vi "Lang Set Desc i.vi"(8 "error in (no error)":errorcluster, 10 "i":T1, 11 "LF2R IDE in":refnum<class "Main Panel.lvclass">) -> (0 "error out":errorcluster, 3 "LF2R IDE out":refnum<class "Main Panel.lvclass">)   [LabVIEW 2018, in "Framework.lvlib" / "Framework.lvclass"]
uses:
  Framework/Framework/Framework.lvclass
  Main Panel.lvclass
  D:/project/hobby/LabVIEW/LF2R/LabVIEW/Source/Actor/Framework/Framework/Framework.lvclass
  C:/Program Files (x86)/National Instruments/LabVIEW 2018/vi.lib/MGI/Panel Manager/Panel Actor/Panel Actor/Panel Actor.lvclass
  C:/Program Files (x86)/National Instruments/LabVIEW 2018/vi.lib/MGI/Monitored Actor/Monitored Actor/Monitored Actor/Monitored Actor.lvclass
  C:/Program Files (x86)/National Instruments/LabVIEW 2018/vi.lib/ActorFramework/Actor/Actor.lvclass
  Const Lang Property.ctl
  Const UI Desc Frame i.ctl
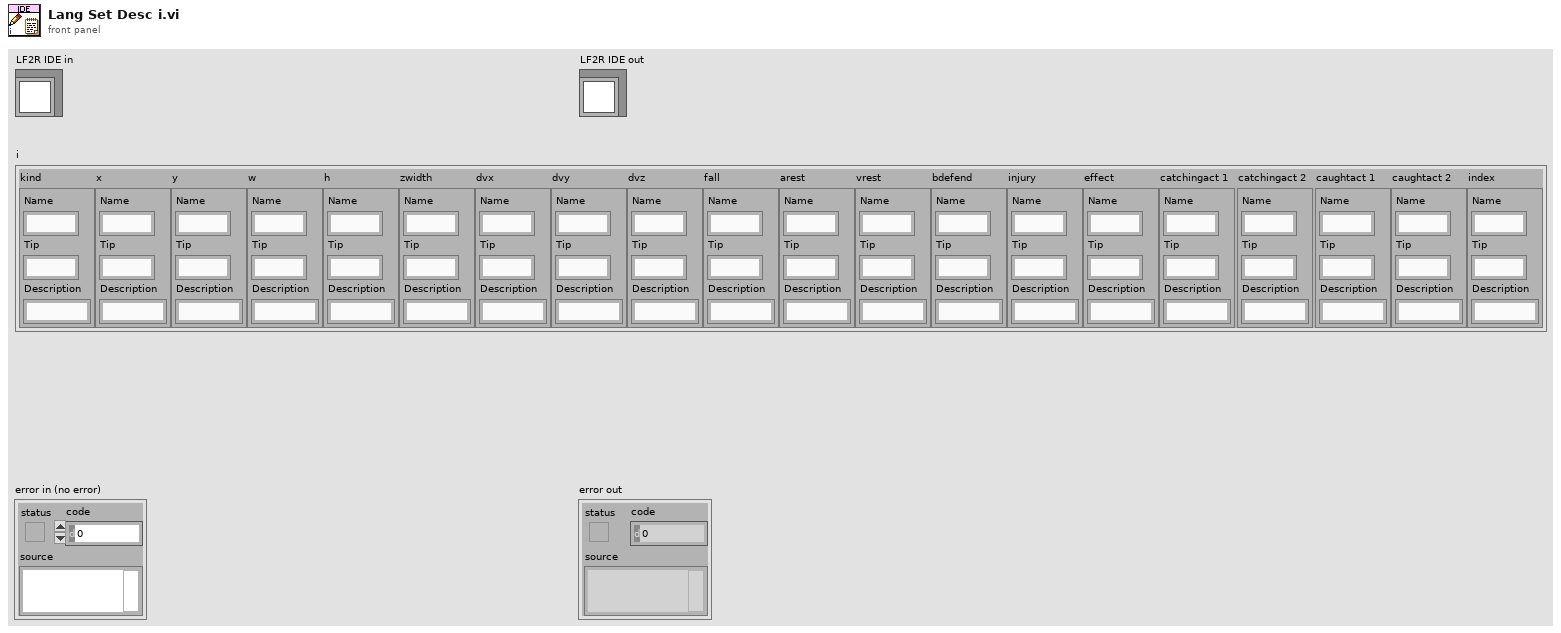
[diagram p1: front panel]
types:
  T1 = typedef "Framework.lvlib/Framework.lvclass/Const UI Desc Frame i.ctl" = cluster{"kind":T2, "x":T2, "y":T2, "w":T2, "h":T2, "zwidth":T2, "dvx":T2, "dvy":T2, "dvz":T2, "fall":T2, "arest":T2, "vrest":T2, "bdefend":T2, "injury":T2, "effect":T2, "catchingact 1":T2, "catchingact 2":T2, "caughtact 1":T2, "caughtact 2":T2, "index":T2}
  T2 = typedef "Framework.lvlib/Framework.lvclass/Const Lang Property.ctl" = cluster{"Name":string, "Tip":string, "Description":string}
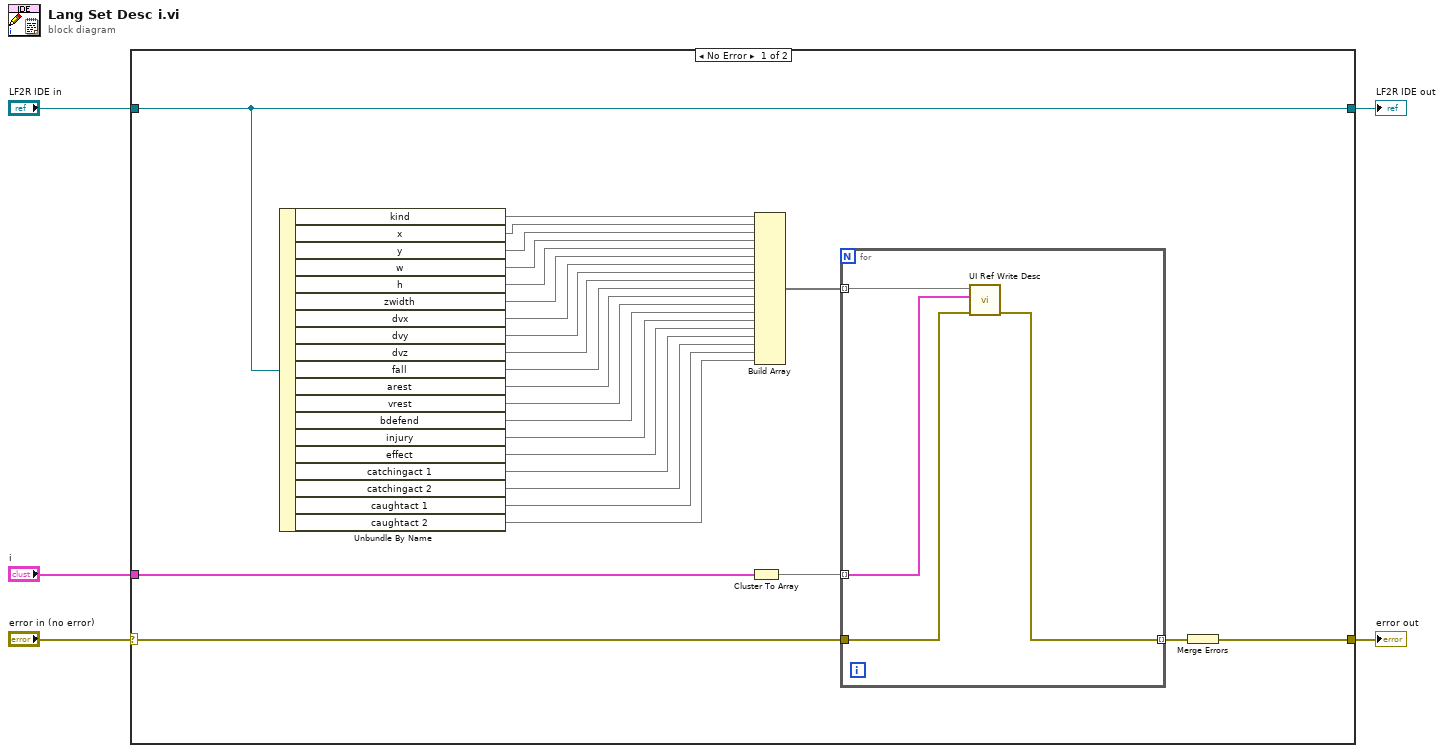
[diagram p0: block diagram]
diagram:
  n1 = case shown="No Error" "error in (no error)" {
    selector: "error in (no error)" -> [w27 w37]
    tunnel: [w25 w37] -> w4
    tunnel: [w31 w36] -> w2
    tunnel: "LF2R IDE in" -> [w31 w36]
    tunnel: "i" -> [w29 _]
    frame No Error {
      n2 = Unbundle By Name(w31) -> ("kind"=w24, "x"=w23, "y"=w22, "w"=w21, "h"=w20, "zwidth"=w19, "dvx"=w18, "dvy"=w17, "dvz"=w16, "fall"=w15, "arest"=w14, "vrest"=w13, "bdefend"=w12, "injury"=w11, "effect"=w10, "catchingact 1"=w9, "catchingact 2"=w8, "caughtact 1"=w7, "caughtact 2"=w6)
      n3 = Cluster To Array(cluster=w29) -> (array=w28:T2[])
      n4 = Build Array(w24, w23, w22, w21, w20, w19, w18, w17, w16, w15, w14, w13, w12, w11, w10, w9, w8, w7, w6) -> (w30:void[])
      n5 = for {
        tunnel: w30 -> [w32] mode=indexing
        tunnel: w28 -> [w35] mode=indexing
        tunnel: w27 -> [w34]
        tunnel: [w33] -> w26 mode=indexing
        n6 = call "UI Ref Write Desc.vi"("error in (no error)"=w34, "UI Property"=w35, "UI Ref"=w32) -> ("error out"=w33:errorcluster)  [unwired: 8 in]
      }
      n7 = Merge Errors(w26) -> (w25:errorcluster)
    }
    frame Error {
    }
  }
  "error out" <- w4
  "LF2R IDE out" <- w2
